vi "Set Sensor Glue Gap.vi"() -> ()   [LabVIEW 2020]
uses:
  Classes/Workspace/Fixture Enum.ctl
  Classes/Routine/Routine Enum.ctl
  Classes/Workspace/Fixture.lvclass
  Classes/Routine/Routine.lvclass
  Classes/Controller/I-O/I-O.lvclass
  Classes/Controller/Controller.lvclass
  Classes/Routine/Pick and Place/Pick and Place.lvclass
  Classes/Controller/Motion/Motion.lvclass
  Classes/Controller/Motion/A3200/A3200.lvclass
panel:
  in  "Tool Height":dbl
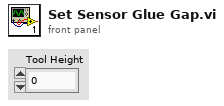
[diagram p1: front panel]
types:
  T1 = typedef "Fixture.lvclass/Fixture Enum.ctl" = enum16{"Assembly Tray", "Syringe Space", "Component", "Pick Up Tool", "Current Position"}
  T2 = typedef "Routine.lvclass/Routine Enum.ctl" = enum16{"Primary Pick Up", "Pick Up All", "Put Down Secondary", "Put Down All", "Release Syringe", "Secondary Pick Up", "Secure Syringe", "Dispense on Plate", "Dispense on Kapton", "Dispense on Sensor"}
  T3 = typedef "Controller.lvclass/Controllers.ctl" = cluster{"I-O.lvclass":refnum<class "I-O.lvclass">, "Gantry":refnum<k24>, "Dispenser":refnum<visa-resource-name>}
  T4 = typedef "Fixture.lvclass/Workspace.ctl" = cluster{"XYZTheta":dbl[], "Workspace Valve":i32, "Workspace Sensor":i32}
  T5 = typedef "I-O.lvclass/Pin Map.ctl" = cluster{"Region Valves":i32[], "Extra Valves":dbl[][][], "Tool Primary Valve":i32, "Tool Secondary Valve":i32, "Region Sensors":i32[], "Extra Sensors":dbl[][][], "Tool Primary Sensor":dbl, "Tool Secondary Sensor":dbl, "Compression Sensor":dbl, "5V":i32, "Dispenser Sensor":dbl}
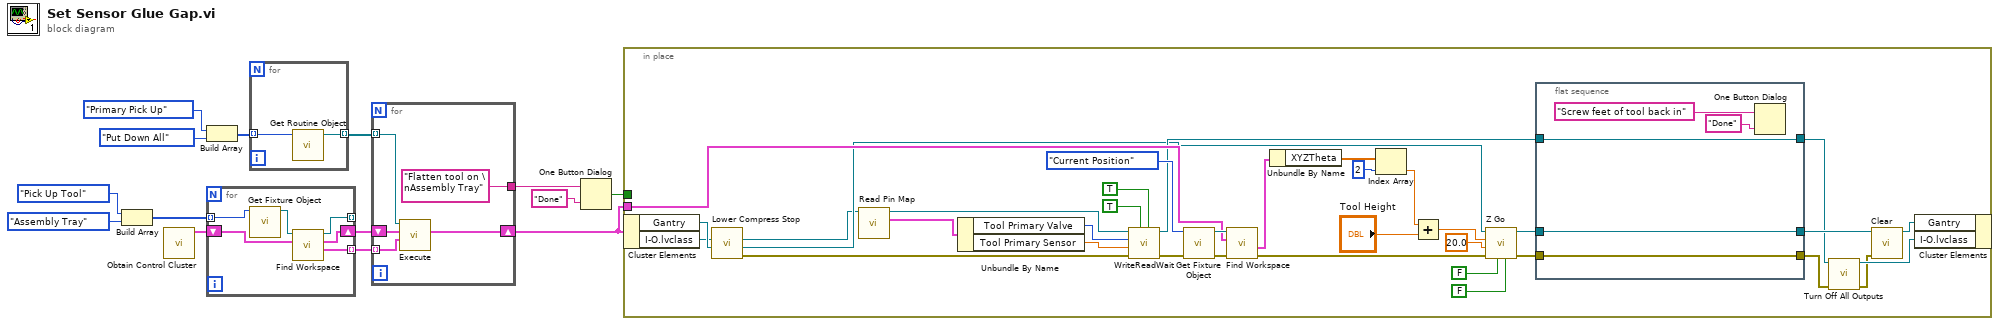
[diagram p0: block diagram]
diagram:
  n1 = Build Array(Fixture_Enum."Pick Up Tool" ("Fixture"), Fixture_Enum."Assembly Tray" ("Fixture")) -> (w5:T1[])
  n2 = call "Obtain Control Cluster.vi"() -> ("Control Out"=w4:T3)  [unwired: 11 in]
  n3 = Build Array(Routine_Enum."Primary Pick Up" ("Routine"), Routine_Enum."Put Down All" ("Routine")) -> (w12:T2[])
  n4 = for {
    tunnel: w5 -> [w20] mode=indexing
    tunnel: [w19] -> _ mode=indexing
    shift-right: [w17] -> w3
    shift-left: w4 -> [w18]
    tunnel: [w16] -> w2 mode=indexing
    n5 = call "Get Fixture Object.vi"("Fixture"=w20) -> ("Workspace.lvclass"=w15:refnum<class "Fixture.lvclass">)  [unwired: 8 in, 2 out]
    n6 = call-dynamic "Find Workspace.vi"("Control In"=w18, "Workspace In"=w15) -> (1:"Workspace Out"=w16:T4, "Control Out"=w17:T3, 3:"Workspace Out"=w19:refnum<class "Fixture.lvclass">)  [unwired: 6 in, 1 out]
  }
  n7 = for {
    tunnel: w12 -> [w22] mode=indexing
    tunnel: [w21] -> w11 mode=indexing
    n8 = call "Get Routine Object.vi"("Routine"=w22) -> ("Routine out"=w21:refnum<class "Routine.lvclass">)  [unwired: 9 in, 1 out]
  }
  n9 = for {
    shift-right: [w25] -> w1
    shift-left: w3 -> [w26]
    tunnel: w11 -> [w27] mode=indexing
    tunnel: ["Flatten tool on \nAssembly Tray"] -> w10
    tunnel: w2 -> [w23] mode=indexing
    n10 = call-dynamic "Execute.vi"("Workspace"=w23, "Control In"=w26, "Routine in"=w27) -> ("Control Out"=w25:T3)  [unwired: 6 in, 2 out]
  }
  n11 = One Button Dialog(message=w10, button name ("OK")="Done") -> (true=w8:bool)
  n12 = in-place {
    in-place-border: w8 -> [_]
    in-place-border: w1 -> [w52]
    n13 = in-place-cluster #1(w1) -> ("Gantry"=w56:refnum<k24>, "I-O.lvclass"=w55:refnum<class "I-O.lvclass">)
    n14 = call "Lower Compress Stop.vi"("Gantry In"=w56, "I-O.lvclass"=w55) -> ("error out"=w42:errorcluster, "Gantry Out"=w33:refnum<k24>, "I-O out"=w30:refnum<class "I-O.lvclass">)  [unwired: 6 in, 1 out]
    n15 = call-dynamic "Read Pin Map.vi"("I-O in"=w30) -> ("Pin Map 2"=w32:T5, "I-O out"=w31:refnum<class "I-O.lvclass">)  [unwired: 8 in, 1 out]
    n16 = Unbundle By Name(w32) -> ("Tool Primary Valve"=w46:i32, "Tool Primary Sensor"=w45:dbl)
    n17 = call "WriteReadWait.vi"("Read Value"=TRUE, "Write Value"=TRUE, "error in (no error)"=w42, "Read"=w45, "Write"=w46, "I-O in"=w31) -> ("error out"=w41:errorcluster, "I-O out"=w40:refnum<class "I-O.lvclass">)  [unwired: 4 in]
    n18 = call "Get Fixture Object.vi"("error in (no error)"=w41, "Fixture"=Fixture_Enum."Current Position") -> ("error out"=w47:errorcluster, "Workspace.lvclass"=w53:refnum<class "Fixture.lvclass">)  [unwired: 7 in, 1 out]
    n19 = call-dynamic "Find Workspace.vi"("Error In"=w47, "Control In"=w52, "Workspace In"=w53) -> ("Error Out"=w36:errorcluster, "Workspace Out"=w51:T4)  [unwired: 5 in, 2 out]
    n20 = Unbundle By Name(w51) -> ("XYZTheta"=w50:dbl[])
    n21 = Index Array(array=w50, index=2) -> (element=w48:dbl)
    n22 = Add(x=w48, y="Tool Height") -> (x+y=w38:dbl)
    n23 = call "Z Go.vi"("Increment"=FALSE, "Return Immediately"=FALSE, "error in (no error)"=w36, "Speed In"=20.0 ("Setting Speed"), "Position In"=w38, "Gantry In"=w33) -> ("error out"=w35:errorcluster, "Gantry Out"=w34:refnum<k24>)  [unwired: 2 in, 2 out]
    n24 = flat-sequence {
      tunnel: w34 -> [w64]
      tunnel: w35 -> [w66]
      tunnel: [w66] -> w61
      tunnel: [w64] -> w58
      tunnel: w40 -> [w63]
      tunnel: [w63] -> w39
      frame #0 {
        n25 = One Button Dialog(message="Screw feet of tool back in", button name ("OK")="Done") -> ()  [unwired: 1 out]
      }
    }
    n26 = call-dynamic "Turn Off All Outputs.vi"("error in (no error)"=w61, "I-O in"=w39) -> ("error out"=w59:errorcluster, "I-O out"=w60:refnum<class "I-O.lvclass">)  [unwired: 8 in]
    n27 = call "Clear.vi"("error in (no error)"=w59, "Gantry In"=w58) -> ("Gantry Out"=w57:refnum<k24>)  [unwired: 8 in, 1 out]
    n28 = in-place-cluster #1("Gantry"=w57, "I-O.lvclass"=w60) -> ()  [unwired: 1 out]
  }
